vi "svc_Exponential Average (1 Ch) (DBL).vi"(10 "normalized time constant (0 = use array length)":dbl, 11 "x":dbl[](array[numeric])) -> (3 "exponential average":dbl=nan)   [LabVIEW 2017]
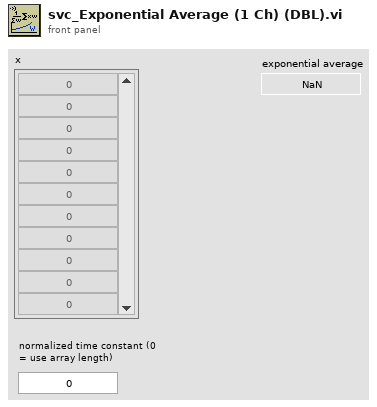
[diagram p1: front panel]
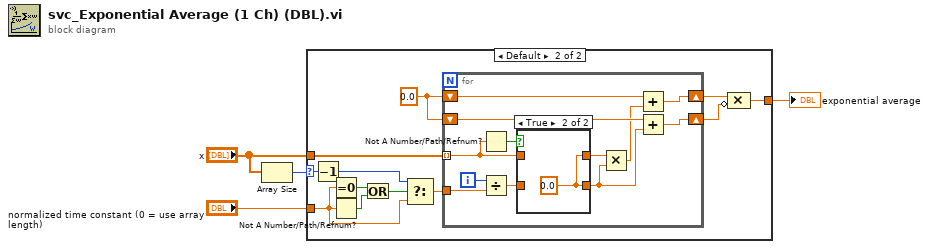
[diagram p0: block diagram]
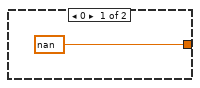
[diagram p2: hidden frame]
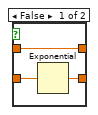
[diagram p3: hidden frame]
diagram:
  n1 = Array Size(array="x") -> (size(s)=w1:i32)
  n2 = case shown="Default" w1 {
    selector: w1 -> [_ w11]
    tunnel: [nan w14] -> w4
    tunnel: "x" -> [_ w13]
    tunnel: "normalized time constant (0 = use array length)" -> [_ w9]
    frame 0 {
    }
    frame Default {
      w17 = 0.0
      n3 = Decrement(x=w11) -> (x-1=w10:i32)
      n4 = Equal To 0?(x=w9) -> (x = 0?=w7:bool)
      n5 = Not A Number/Path/Refnum?(number/path/refnum=w9) -> (NaN/Path/Refnum?=w8:bool)
      n6 = Or(x=w7, y=w8) -> (x .or. y?=w6:bool)
      n7 = Select(t=w10, s=w6, f=w9) -> (s? t:f=w12:dbl)
      n8 = for {
        tunnel: w13 -> [w18] mode=indexing
        tunnel: w12 -> [w28]
        shift-right: [w22] -> w15
        shift-left: w17 -> [w26]
        shift-right: [w24] -> w16
        shift-left: w17 -> [w25]
        i -> [w29]
        n9 = Not A Number/Path/Refnum?(number/path/refnum=w18) -> (NaN/Path/Refnum?=w20:bool)
        n10 = Divide(x=w29, y=w28) -> (x/y=w27:dbl)
        n11 = case shown="True" w20 {
          tunnel: w27 -> [w32 _]
          tunnel: [w31 w33] -> w21
          tunnel: [w30 w33] -> w19
          tunnel: w18 -> [w30 _]
          frame False {
            n12 = Exponential(1:w32) -> (0:w31:dbl)
          }
          frame True {
            w33 = 0.0
          }
        }
        n13 = Multiply(x=w19, y=w21) -> (x*y=w23:dbl)
        n14 = Add(x=w26, y=w23) -> (x+y=w22:dbl)
        n15 = Add(x=w25, y=w21) -> (x+y=w24:dbl)
      }
      n16 = Compound Arithmetic op=MULTIPLY(w15, invert w16) -> (w14:dbl)
    }
  }
  "exponential average" <- w4
